vi "lvEtherbone.error_handler.vi"(2 "eb_status":T1 items=["EB_SUCCESS"=1, "EB_OK"=0, "EB_FAIL"=-1, "EB_ADDRESS"=-2, "EB_WIDTH"=-3, "EB_OVERFLOW"=-4, "EB_ENDIAN"=-5, "EB_BUSY"=-6, "EB_TIMEOUT"=-7, "EB_OOM"=-8, "EB_ABI"=-9, "EB_SEGFAULT"=-10], 5 "error in":errorcluster) -> (19 "error out":errorcluster)   [LabVIEW 2012, in "lvEtherbone.lvlib"]
doc: "Builds an error cluster depending on \"eb_status\" and call chain"
uses:
  lvEtherbone.lvlib
  lvEtherbone.lveb_status_t.ctl
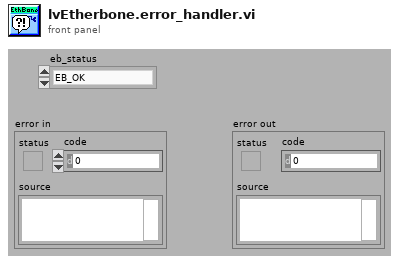
[diagram p1: front panel]
types:
  T1 = typedef "lvEtherbone.lvlib/lvEtherbone.lveb_status_t.ctl" = i32
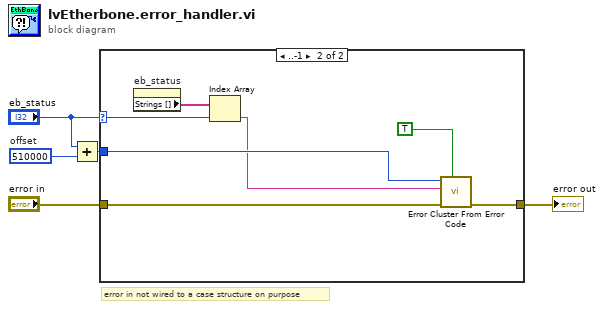
[diagram p0: block diagram]
diagram:
  w2 = 510000  # offset
  # "error in not wired to a case structure on purpose"
  n1 = Add(x="eb_status", y=w2) -> (x+y=w1:T1)
  n2 = case shown="..-1" "eb_status" {
    selector: "eb_status" -> [_ w8]
    tunnel: "error in" -> [w6 w11]
    tunnel: [w6 w12] -> w5
    tunnel: w1 -> [_ w10]
    frame 0, Default {
    }
    frame ..-1 {
      n3 = property on="eb_status" class="Ring (strict)"() -> ("Strings []"=w9:string[])  [unwired: 2 in, 2 out]
      n4 = Index Array(array=w9, index=w8) -> (element=w7:string)
      n5 = call <vilib>:"Error Cluster From Error Code.vi"("show call chain? (False)"=TRUE, "error in (no error)"=w11, "error message (\"\")"=w7, "error code (0)"=w10) -> ("error out"=w12:errorcluster)  [unwired: 5 in]
    }
  }
  "error out" <- w5
